vi "Base.Device.SetDeviceState.vi"(8 "error in (no error)":errorcluster, 10 "Device State":variant, 11 "Device.Simulation in":refnum<class "Device.Simulation.lvclass">) -> (0 "error out":errorcluster, 3 "Device.Simulation out":refnum<class "Device.Simulation.lvclass">)   [LabVIEW 2019, in "Device.Simulation.lvlib" / "Device.Simulation.lvclass"]
uses:
  Device.Simulation.lvclass
  state--cluster.ctl
  Device.Simulation.lvclass/Device.Simulation.ctl
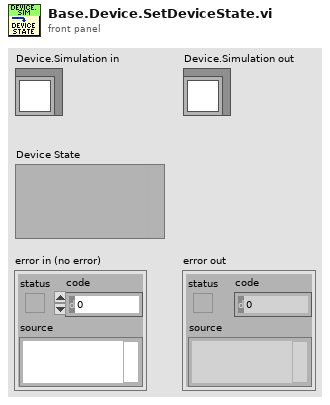
[diagram p1: front panel]
types:
  T1 = typedef "Device.Simulation.lvlib/Device.Simulation.lvclass/state--cluster.ctl" = cluster{"A1":dbl, "A2":dbl, "A3":dbl, "D1":bool, "D2":bool, "D3":bool}
  T2 = typedef "Device.Simulation.lvlib/Device.Simulation.lvclass/privateData--reference.ctl" = refnum<data-value>
  T3 = typedef "Device.Simulation.lvlib/Device.Simulation.lvclass/privateData--cluster.ctl" = cluster{"config":T4, "state":T1}
  T4 = typedef "Device.Simulation.lvlib/Device.Simulation.lvclass/config--cluster.ctl" = cluster{"Name":string, "Time to Connect (ms)":u32, "Time to Check Connection (ms)":u32, "Time to Disconnect (ms)":u32, "Time to Read State (ms)":u32}
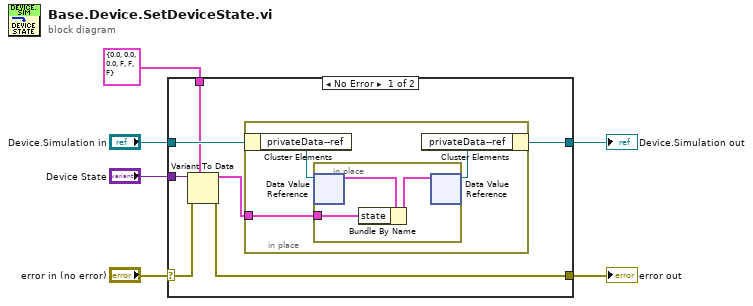
[diagram p0: block diagram]
diagram:
  n1 = case shown="No Error" "error in (no error)" {
    selector: "error in (no error)" -> [w8 w21]
    tunnel: [w7 w21] -> w4
    tunnel: [w12 w20] -> w5
    tunnel: "Device.Simulation in" -> [w13 w20]
    tunnel: "Device State" -> [w11 _]
    tunnel: T1 {"A1"=0.0, "A2"=0.0, "A3"=0.0, "D1"=FALSE, "D2"=FALSE, "D3"=FALSE} ("state") -> [w10 _]
    frame No Error {
      n2 = Variant To Data(error in=w8, type=w10, Variant=w11) -> (data=w9:T1, error out=w7:errorcluster)
      n3 = in-place {
        in-place-border: w9 -> [w14]
        n4 = in-place-cluster #1(w13) -> ("privateData--ref"=w16:T2)
        n5 = in-place {
          in-place-border: w14 -> [w17]
          n6 = in-place-dvr #2(w16) -> (w19:T3)  [unwired: 1 out]
          n7 = Bundle By Name(cluster=w19, "state"=w17) -> (w18:T3)
          n8 = in-place-dvr #2(w18) -> (w15:T2)  [unwired: 1 out]
        }
        n9 = in-place-cluster #1("privateData--ref"=w15) -> (w12:refnum<class "Device.Simulation.lvclass">)
      }
    }
    frame Error {
    }
  }
  "error out" <- w4
  "Device.Simulation out" <- w5
